vi "FindLowstVarDimNamePari.vi"(1 "dims":cluster{"name":string, "size":u64}[](array[cluster]), 2 "vars":T1(array[cluster])) -> (0 "var-lowst-dim name pair":cluster{"name":string, "name":string}[](array[cluster]))   [LabVIEW 2016]
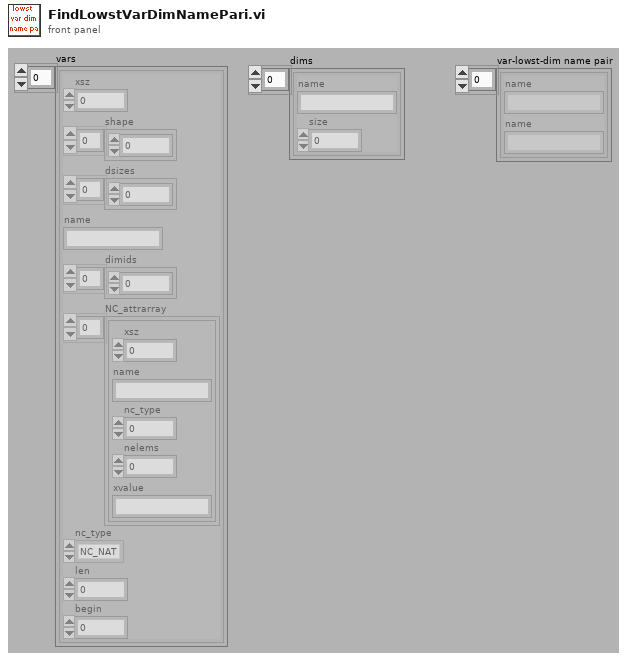
[diagram p1: front panel]
types:
  T1 = cluster{"xsz":u64, "shape":u64[], "dsizes":u64[], "name":string, "dimids":u64[], "NC_attrarray":cluster{"xsz":u64, "name":string, "nc_type":u16, "nelems":u64, "xvalue":string}[], "nc_type":enum16{"NC_NAT", "NC_BYTE", "NC_CHAR", "NC_SHORT", "NC_INT", "NC_FLOAT", "NC_DOUBLE"}, "len":u64, "begin":u64}[]
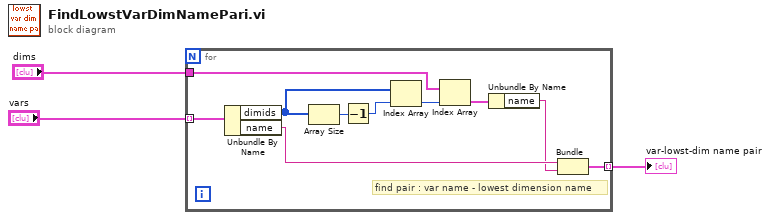
[diagram p0: block diagram]
diagram:
  n1 = for {
    tunnel: "vars" -> [w13] mode=indexing
    tunnel: [w5] -> w1 mode=indexing
    tunnel: "dims" -> [w4]
    # "find pair : var name - lowest dimension name"
    n2 = Unbundle By Name(w13) -> ("dimids"=w11:u64[], "name"=w7:string)
    n3 = Array Size(array=w11) -> (size(s)=w12:i32)
    n4 = Decrement(x=w12) -> (x-1=w10:i32)
    n5 = Index Array(array=w11, index=w10) -> (element=w9:u64)
    n6 = Index Array(array=w4, index=w9) -> (element=w8:cluster{"name":string, "size":u64})
    n7 = Unbundle By Name(w8) -> ("name"=w6:string)
    n8 = Bundle("name"=w7, "name"=w6) -> (w5:cluster{"name":string, "name":string})  [unwired: 1 out]
  }
  "var-lowst-dim name pair" <- w1
